vi "CTFTMain_Menu.vi"() -> ()   [LabVIEW 2009]
uses:
  <vilib>/Platform/browser.llb/Open URL in Default Browser (string).vi
panel:
  in  "Exit":bool
  in  "Select Option":string(tree)="Aliasing"
  # "Signal Processing Lab\n       LabVIEW"
  # "Powered by\n\n                                        http://www.ni.com"
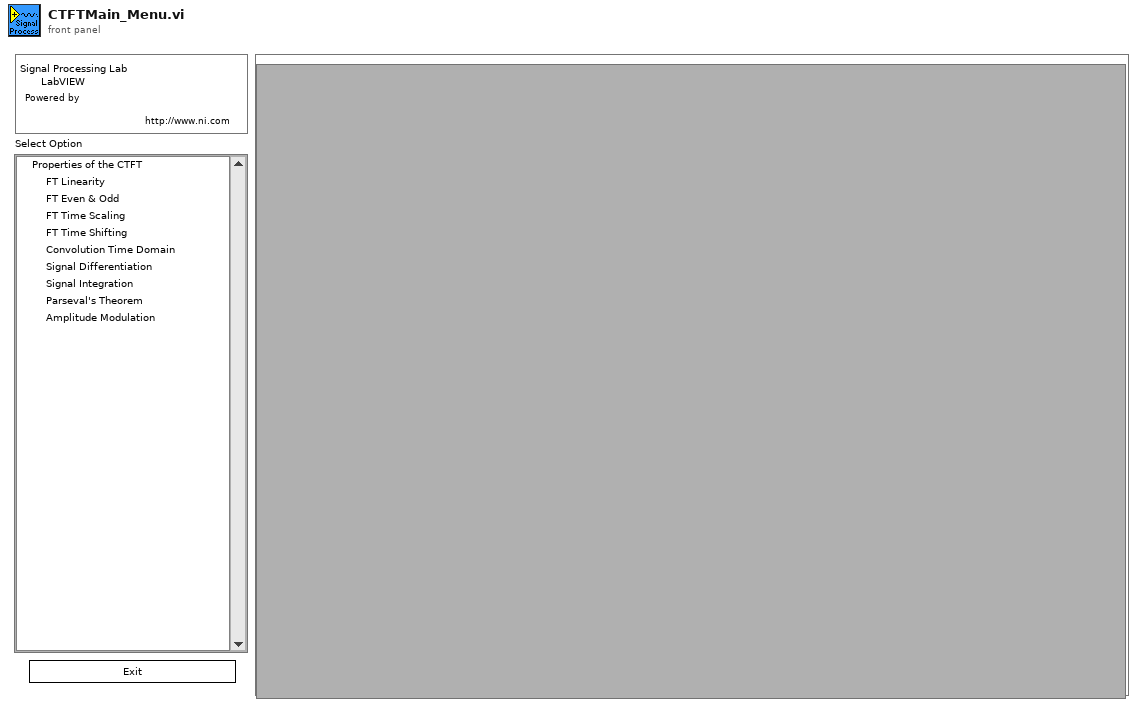
[diagram p1: front panel]
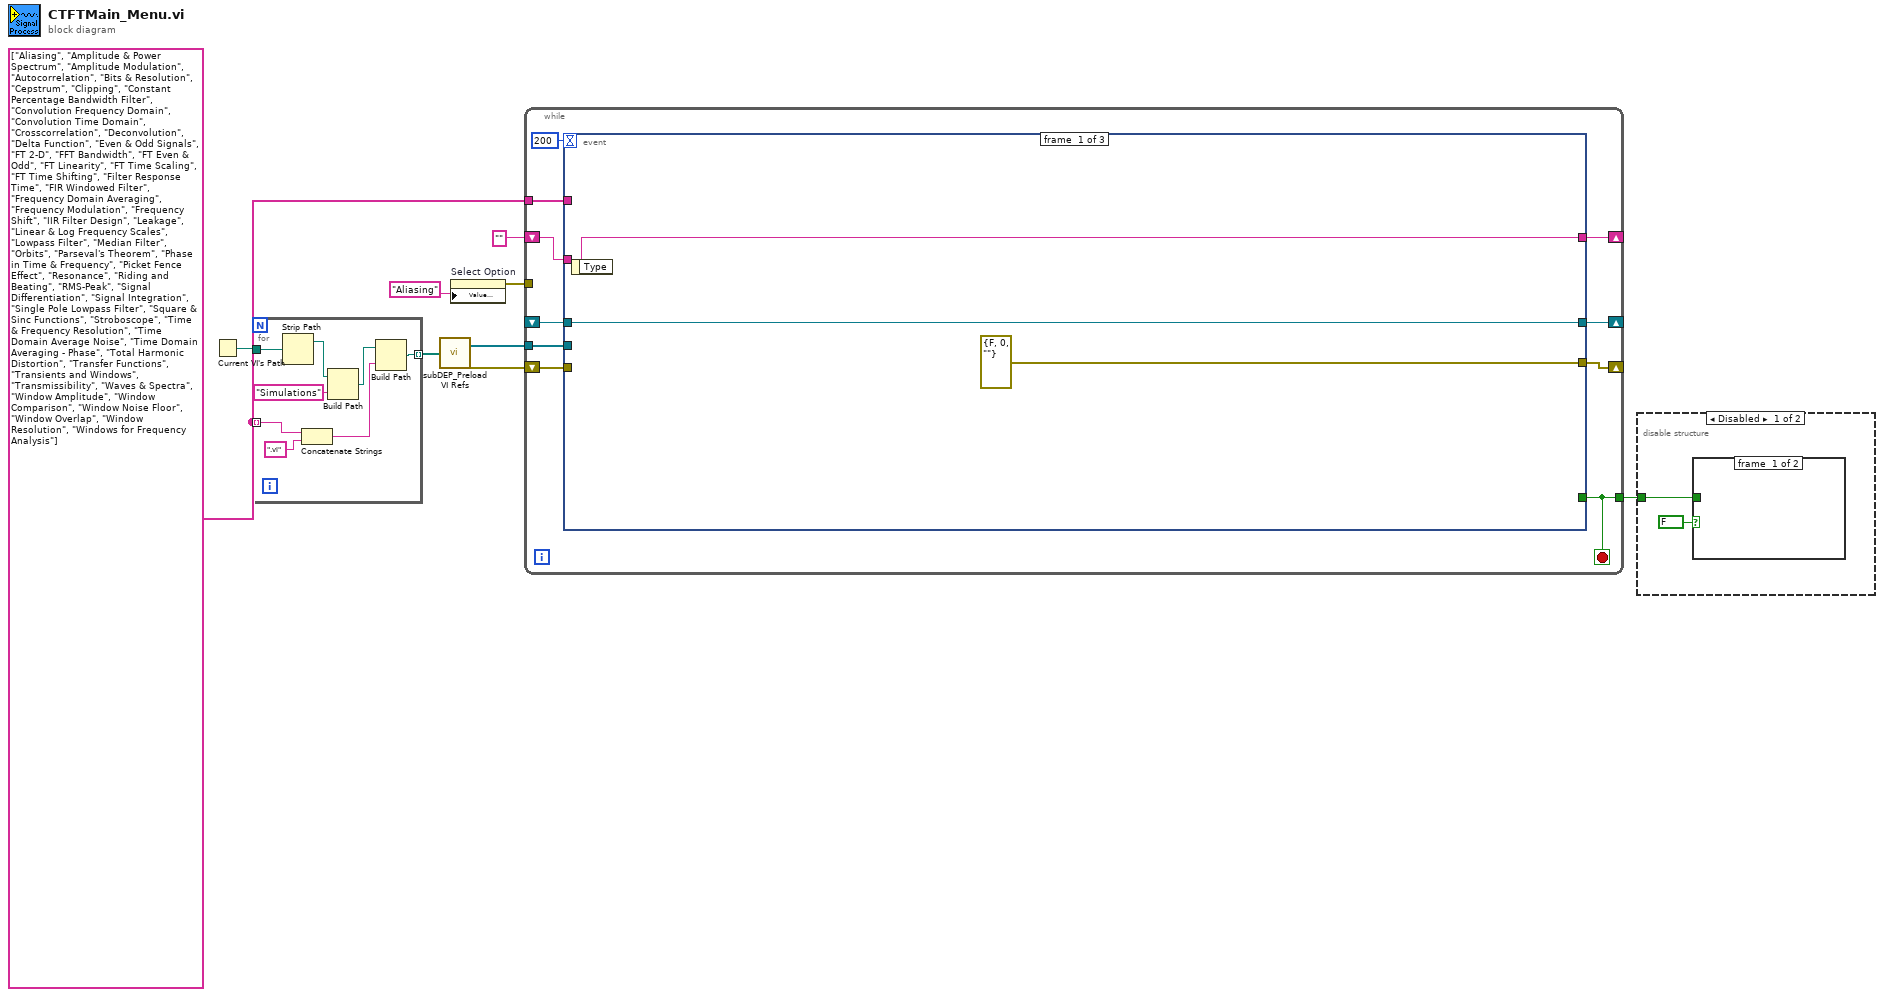
[diagram p0: block diagram]
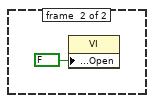
[diagram p2: hidden frame]
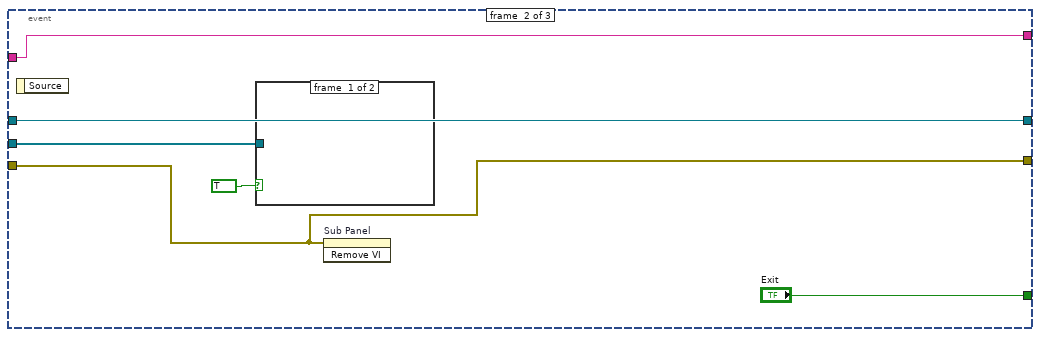
[diagram p4: hidden frame]
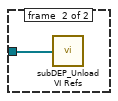
[diagram p5: hidden frame]
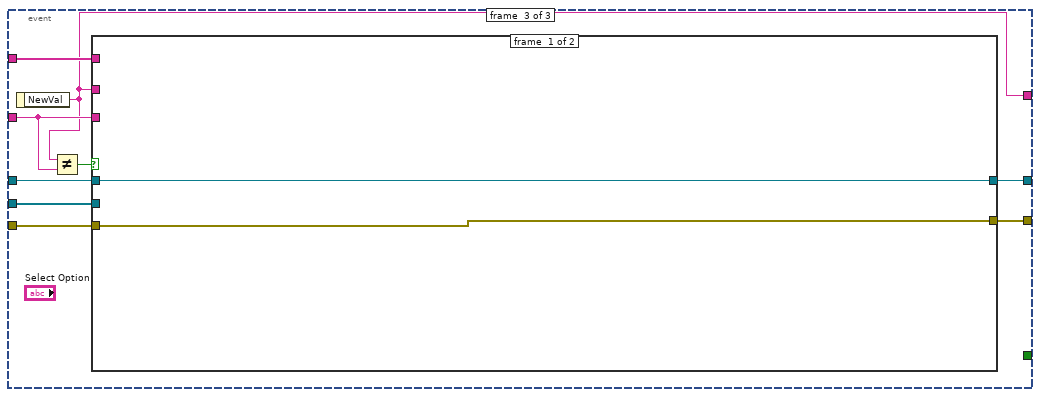
[diagram p6: hidden frame]
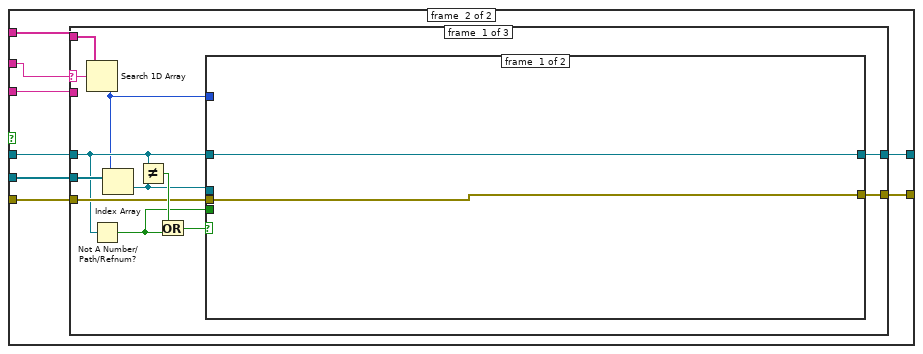
[diagram p7: hidden frame]
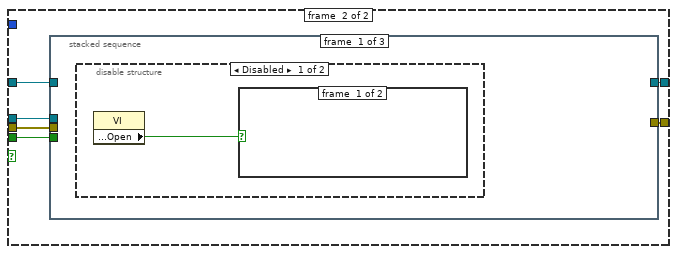
[diagram p8: hidden frame]
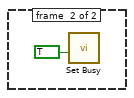
[diagram p9: hidden frame]
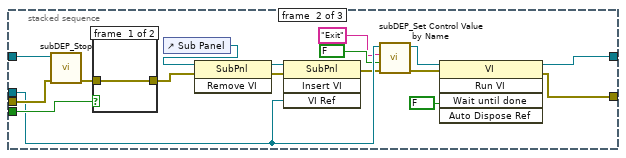
[diagram p11: hidden frame]
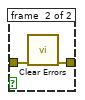
[diagram p12: hidden frame]
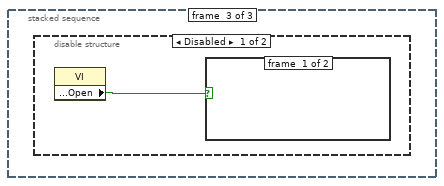
[diagram p13: hidden frame]
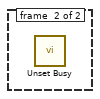
[diagram p14: hidden frame]
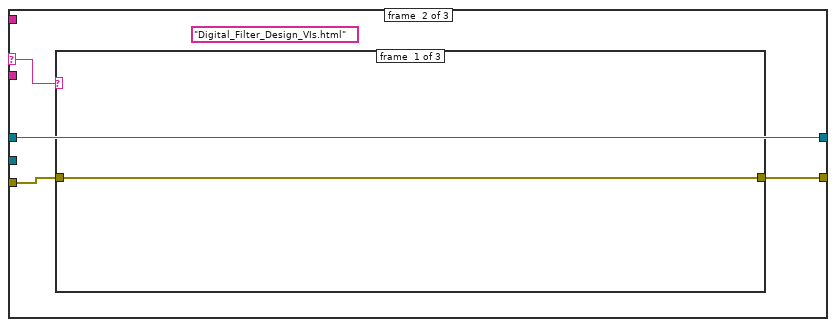
[diagram p16: hidden frame]
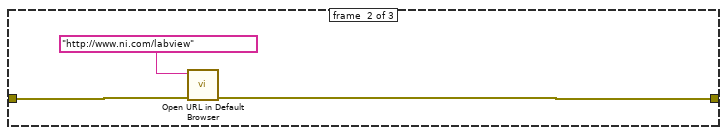
[diagram p17: hidden frame]
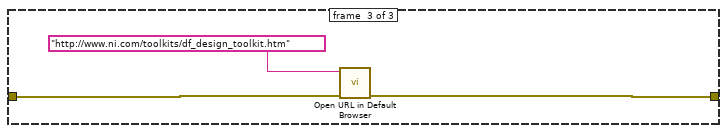
[diagram p18: hidden frame]
diagram:
  w3 = string[] ["Aliasing", "Amplitude & Power Spectrum", "Amplitude Modulation", "Autocorrelation", "Bits & Resolution", "Cepstrum", "Clipping", "Constant Percentage Bandwidth Filter", "Convolution Frequency Domain", "Convolution Time Domain", "Crosscorrelation", "Deconvolution", "Delta Function", "Even & Odd Signals", "FT 2-D", "FFT Bandwidth", "FT Even & Odd", "FT Linearity", "FT Time Scaling", "FT Time Shifting", "Filter Response Time", "FIR Windowed Filter", "Frequency Domain Averaging", "Frequency Modulation", "Frequency Shift", "IIR Filter Design", "Leakage", "Linear & Log Frequency Scales", "Lowpass Filter", "Median Filter", "Orbits", "Parseval's Theorem", "Phase in Time & Frequency", "Picket Fence Effect", "Resonance", "Riding and Beating", "RMS-Peak", "Signal Differentiation", "Signal Integration", "Single Pole Lowpass Filter", "Square & Sinc Functions", "Stroboscope", "Time & Frequency Resolution", "Time Domain Average Noise", "Time Domain Averaging - Phase", "Total Harmonic Distortion", "Transfer Functions", "Transients and Windows", "Transmissibility", "Waves & Spectra", "Window Amplitude", "Window Comparison", "Window Noise Floor", "Window Overlap", "Window Resolution", "Windows for Frequency Analysis"] ("Array")
  n1 = Current VI's Path() -> (path=w5:path)
  n2 = for {
    tunnel: w5 -> [w17]
    tunnel: w3 -> [w16] mode=indexing
    tunnel: [w13] -> w4 mode=indexing
    n3 = Strip Path(path=w17) -> (stripped path=w11:path)  [unwired: 1 out]
    n4 = Concatenate Strings(w16, ".vi" ("regular expression")) -> (w14:string)
    n5 = Build Path(base path=w11, name or relative path="Simulations") -> (appended path=w10:path)
    n6 = Build Path(base path=w10, name or relative path=w14) -> (appended path=w13:path)
  }
  n7 = call "subDEP_Preload VI Refs.vi"("VI Paths"=w4) -> ("VI Refs"=w8:refnum<vi>[], "error out"=w7:errorcluster)
  n8 = property on="Select Option" class="Tree (strict)"("Value (Signaling)"="Aliasing") -> (error out=w9:errorcluster)  [unwired: 2 in, 1 out]
  n9 = while {
    tunnel: w3 -> [w26]
    tunnel: w8 -> [w25]
    tunnel: w9 -> [_]
    shift-right: [w22] -> _
    shift-left: _ -> [w24]
    shift-right: [w21] -> _
    shift-left: w7 -> [w23]
    tunnel: [w20] -> w6
    shift-right: [w19] -> _
    shift-left: "" -> [w18]
    stop <- w20 stop-if-true
    n10 = event shown="[1] \"Exit\": Value Change" {
      selector: _ -> [_ _ _]
      dyn-events: _ -> [_ _ _]
      timeout: 200 -> [_ _ _]
      tunnel: w26 -> [_ _ w41]
      tunnel: w25 -> [_ w35 w46]
      tunnel: [_ "Exit" _] -> w20
      tunnel: w24 -> [w29 w34 w45]
      tunnel: w23 -> [_ w31 w44]
      tunnel: [w29 w34 w43] -> w22
      tunnel: [errorcluster {"status"=FALSE, "code"=0, "source"=""} ("error out") w31 w42] -> w21
      tunnel: [w28 w33 w38] -> w19
      tunnel: w18 -> [w28 w33 w40]
      event #0 {
        n11 = event-data() -> ()  [unwired: 1 in, 1 out]
      }
      event #1 {
        n12 = event-data() -> ()  [unwired: 1 in, 1 out]
        n13 = case shown="True" TRUE {
          tunnel: w35 -> [_ w37]
          frame #0 {
          }
          frame #1 {
            n14 = call "subDEP_Unload VI Refs.vi"("VI Refs"=w37) -> ()
          }
        }
        n15 = invoke on="Sub Panel" class="SubPanel" method="Remove VI"(error in=w31) -> ()  [unwired: 2 in, 3 out]
      }
      event #2 {
        n16 = event-data() -> ("NewVal"=w38:string)  [unwired: 1 in]
        n17 = Not Equal?(x=w38, y=w40) -> (x != y?=w39:bool)
        n18 = case shown="True" w39 {
          tunnel: w46 -> [_ w56]
          tunnel: w45 -> [w47 w55]
          tunnel: w44 -> [w48 w54]
          tunnel: [w47 w53] -> w43
          tunnel: [w48 w52] -> w42
          tunnel: w41 -> [_ w51]
          tunnel: w38 -> [_ w49]
          tunnel: w40 -> [_ w50]
          frame #0 {
          }
          frame #1 {
            n19 = case shown="\"False\", Default" w49 {
              selector: w49 -> [w58 w102 _]
              tunnel: w56 -> [w68 _ _]
              tunnel: w55 -> [w61 w103 w112]
              tunnel: w54 -> [w64 w101 w111]
              tunnel: [w63 w103 w112] -> w53
              tunnel: [w62 w100 w111] -> w52
              tunnel: w51 -> [w59 _ _]
              tunnel: w50 -> [_ _ _]
              frame #0 {
                n20 = Search 1D Array(1D array=w59, element=w58) -> (index of element=w57:i32)  [unwired: 1 in]
                n21 = Not A Number/Path/Refnum?(number/path/refnum=w61) -> (NaN/Path/Refnum?=w60:bool)
                n22 = Index Array(array=w68, index=w57) -> (element=w65:refnum<vi>)
                n23 = Not Equal?(x=w61, y=w65) -> (x != y?=w67:bool)
                n24 = Or(x=w67, y=w60) -> (x .or. y?=w66:bool)
                n25 = case shown="True" w66 {
                  tunnel: w61 -> [w70 w76]
                  tunnel: w65 -> [_ w73]
                  tunnel: w64 -> [w69 w75]
                  tunnel: w60 -> [_ w74]
                  tunnel: [w70 w71] -> w63
                  tunnel: [w69 w72] -> w62
                  tunnel: w57 -> [_ _]
                  frame #0 {
                  }
                  frame #1 {
                    n26 = stacked-sequence {
                      tunnel: w76 -> [_ w95 _]
                      tunnel: w75 -> [_ w94 _]
                      tunnel: w74 -> [_ w93 _]
                      tunnel: w73 -> [_ w84 _]
                      tunnel: [_ w89 _] -> w72
                      tunnel: [_ w90 _] -> w71
                      frame #0 {
                        n27 = disable-structure shown="Disabled" {
                          frame #0 {
                            n28 = property class="VI"() -> ("Front Panel Window:Open"=w77:bool)  [unwired: 2 in, 2 out]
                            n29 = case shown="True" w77 {
                              frame #0 {
                              }
                              frame #1 {
                                n30 = call <vilib>:"Set Busy.vi"("disable click? (T)"=TRUE) -> ()  [unwired: 9 in, 2 out]
                              }
                            }
                          }
                          frame #1 {
                          }
                        }
                      }
                      frame #1 {
                        n31 = call "subDEP_Stop.vi"("error in (no error)"=w94, "vi refnum in"=w95) -> ("error out"=w92:errorcluster)  [unwired: 8 in, 1 out]
                        n32 = case shown="True" w93 {
                          tunnel: w92 -> [w96 w98]
                          tunnel: [w96 w97] -> w88
                          frame #0 {
                          }
                          frame #1 {
                            n33 = call <vilib>:"Clear Errors.vi"("error in (no error)"=w98) -> ("error out"=w97:errorcluster)  [unwired: 6 in]
                          }
                        }
                        n34 = control-ref of="Sub Panel"() -> (w87:refnum<vi>)
                        n35 = invoke class="SubPnl" method="Remove VI"(reference=w87, error in=w88) -> (reference out=w86:refnum<vi>, error out=w85:errorcluster)  [unwired: 1 in, 1 out]
                        n36 = invoke class="SubPnl" method="Insert VI"(reference=w86, error in=w85, "VI Ref"=w84) -> (error out=w81:errorcluster)  [unwired: 1 in, 3 out]
                        n37 = call "subDEP_Set Control Value by Name.vi"("error in (no error)"=w81, "Value"=FALSE ("Boolean"), "control name"="Exit" ("Control Name"), "vi reference in"=w84) -> ("error out"=w82:errorcluster, "vi reference out"=w83:refnum<vi>)  [unwired: 6 in]
                        n38 = invoke class="VI" method="Run VI"(reference=w83, error in=w82, "Wait until done"=FALSE) -> (reference out=w90:refnum<vi>, error out=w89:errorcluster)  [unwired: 2 in, 3 out]
                      }
                      frame #2 {
                        n39 = disable-structure shown="Disabled" {
                          frame #0 {
                            n40 = property class="VI"() -> ("Front Panel Window:Open"=w99:bool)  [unwired: 2 in, 2 out]
                            n41 = case shown="True" w99 {
                              frame #0 {
                              }
                              frame #1 {
                                n42 = call <vilib>:"Unset Busy.vi"() -> ()  [unwired: 11 in, 1 out]
                              }
                            }
                          }
                          frame #1 {
                          }
                        }
                      }
                    }
                  }
                }
              }
              frame #1 {
                (unwired) "Digital_Filter_Design_VIs.html"
                n43 = case shown="\"Digital Filter Design\\nToolkit for LabVIEW\"" w102 {
                  tunnel: w101 -> [w104 w107 w110]
                  tunnel: [w104 w106 w109] -> w100
                  frame #0 {
                  }
                  frame #1 {
                    n44 = call-poly <vilib>:"Open URL in Default Browser.vi"("error in (no error)"=w107, "URL"="http://www.ni.com/labview") -> ("error out"=w106:errorcluster)  [unwired: 4 in, 1 out]
                  }
                  frame #2 {
                    n45 = call-poly <vilib>:"Open URL in Default Browser.vi"("error in (no error)"=w110, "URL"="http://www.ni.com/toolkits/df_design_toolkit.htm") -> ("error out"=w109:errorcluster)  [unwired: 4 in, 1 out]
                  }
                }
              }
              frame #2 {
              }
            }
          }
        }
      }
    }
  }
  n46 = disable-structure shown="Disabled" {
    disable-tunnel: w6 -> [w114 _]
    frame #0 {
      n47 = case shown="True" FALSE {
        tunnel: w114 -> [_ _]
        frame #0 {
        }
        frame #1 {
          n48 = property class="VI"("Front Panel Window:Open"=FALSE) -> ()  [unwired: 2 in, 2 out]
        }
      }
    }
    frame #1 {
    }
  }
